vi "TestStand - BuildPPLWrapper.vi"(9 "Target":string="My Computer", 10 "BuildSpecification":string, 11 "ProjectPath":path) -> (2 "error out":errorcluster, 3 "Generated files":path[](array[path]))   [LabVIEW 2025]
uses:
  <vilib>/AppBuilder/AB_API_Simple/Build (path).vi
  <vilib>/AppBuilder/AB_API_Simple/NI_App_Builder_API.lvlib
panel:
  in  "error in (no error)":errorcluster
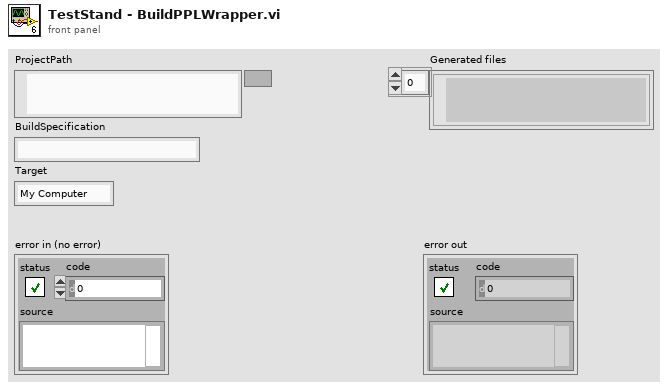
[diagram p1: front panel]
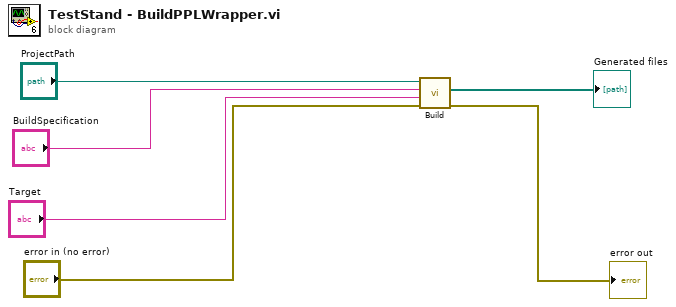
[diagram p0: block diagram]
diagram:
  n1 = call-poly <vilib>:"Build.vi"("error in (no error)"="error in (no error)", "Name of target (My Computer)"="Target", "Name of build specification (if empty: build all)"="BuildSpecification", "Path to project"="ProjectPath") -> ("error out"=→"error out":errorcluster, "Generated files"=→"Generated files":path[])  [unwired: 6 in]
